vi "Curtin1_SelectTemplate.vi"(11 "Settings in":T1={"Name of test"="", "Date"=timestamp(0 s since 1904-01-01), "Location"="", "Template"="", "Soundcard"="", "resolution"=32, "Sampling rate"=48000, "Ch1 Gain "=25.0, "Ch2 Gain"=10.0, "Sample time (s)"=0.3, "Pre-trigger (s)"=0.01, "Hammer Threshold"=10.0, "Positions"=12, "Taps/Position"=5, "Set Names"="", "Freq resolution"=10.0, "Hammer cutoff"=0.0, "Mic cutoff"=0.0, "Double bounce "=0.0, "Hammer Cal"=10.0, "dB Offset"=0.0, "Accel Cal"=10.0, "Vibrometer Cal"=0.0, "Mic Cal"=0.0, "Output"=2, "Voltage Cal"=0.01, "Vibrometer Port"="ASRL27::INSTR", "Range"=4, "High Pass"=2, "Bandwidth"=4, "X Range"=[], "Y Range"=[], "dB Spread"=0.0, "Trigger"=0, "Ch_1"=25, "Ch_2"=25, "flip?"=FALSE, "60Hz"=FALSE, "Time offset"=0.0, "Piezo Cal"=1.0, "Default Notes"=""} {"Ch_2" min=1 step=1; "Ch_1" min=1 max=100 step=1; "Trigger" items=["Hammer (force)", "Self-tap", "Spacebar"]; "Bandwidth" items=["1 kHz"=1, "5 kHz"=5, "10 kHz"=10, "25 kHz"=25, "50 kHz"=50, "100 kHz"=100]; "High Pass" items=["Off", "13 Hz", "104 Hz"]; "Range" items=["10 mm/s"=1, "20 mm/s"=2, "50 mm/s"=5, "100 mm/s"=10, "200 mm/s"=20, "500 mm/s"=50, "1 m/s"=100, "2 m/s"=200]; "Output" items=["Accelerometer", "Speed (from acceleration)", "Microphone", "Vibrometer", "Piezo"]; "Voltage Cal" format="%#_13g"; "Ch2 Gain" format="%#_13g"; "Ch1 Gain" format="%#_13g"; "Double bounce" min=0.0; "Mic cutoff" min=0.0 format="%#_4g"; "Hammer cutoff" min=0.0 format="%#_4g"; "Freq resolution" min=0.0; "Pre-trigger (s)" format="%#_13g"; "Date" format="%<%H:%M\n%d/%m/%y>T"; "resolution" items=["16 bit"=16, "24 bit"=24, "32 bit"=32]; "Sampling rate" items=["22050 samp/s"=22050, "44100 samp/s"=44100, "48000 samp/s"=48000]}) -> (1 "New Template":string, 3 "Settings out":T1={"Name of test"="", "Date"=timestamp(0 s since 1904-01-01), "Location"="", "Template"="", "Soundcard"="", "resolution"=32, "Sampling rate"=48000, "Ch1 Gain "=25.0, "Ch2 Gain"=10.0, "Sample time (s)"=0.3, "Pre-trigger (s)"=0.01, "Hammer Threshold"=10.0, "Positions"=12, "Taps/Position"=5, "Set Names"="", "Freq resolution"=10.0, "Hammer cutoff"=0.0, "Mic cutoff"=0.0, "Double bounce "=0.0, "Hammer Cal"=10.0, "dB Offset"=0.0, "Accel Cal"=10.0, "Vibrometer Cal"=0.0, "Mic Cal"=0.0, "Output"=2, "Voltage Cal"=0.01, "Vibrometer Port"="ASRL27::INSTR", "Range"=4, "High Pass"=2, "Bandwidth"=4, "X Range"=[], "Y Range"=[], "dB Spread"=0.0, "Trigger"=0, "Ch_1"=25, "Ch_2"=25, "flip?"=FALSE, "60Hz"=FALSE, "Time offset"=0.0, "Piezo Cal"=1.0, "Default Notes"=""} {"Ch_2" min=1 step=1; "Ch_1" min=1 max=100 step=1; "Trigger" items=["Hammer (force)", "Self-tap", "Spacebar"]; "Bandwidth" items=["1 kHz"=1, "5 kHz"=5, "10 kHz"=10, "25 kHz"=25, "50 kHz"=50, "100 kHz"=100]; "High Pass" items=["Off", "13 Hz", "104 Hz"]; "Range" items=["10 mm/s"=1, "20 mm/s"=2, "50 mm/s"=5, "100 mm/s"=10, "200 mm/s"=20, "500 mm/s"=50, "1 m/s"=100, "2 m/s"=200]; "Output" items=["Accelerometer", "Speed (from acceleration)", "Microphone", "Vibrometer", "Piezo"]; "Voltage Cal" format="%#_13g"; "Ch2 Gain" format="%#_13g"; "Ch1 Gain" format="%#_13g"; "Double bounce" min=0.0; "Mic cutoff" min=0.0 format="%#_4g"; "Hammer cutoff" min=0.0 format="%#_4g"; "Freq resolution" min=0.0; "Pre-trigger (s)" format="%#_13g"; "Date" format="%<%H:%M\n%d/%m/%y>T"; "resolution" items=["16 bit"=16, "24 bit"=24, "32 bit"=32]; "Sampling rate" items=["22050 samp/s"=22050, "44100 samp/s"=44100, "48000 samp/s"=48000]})   [LabVIEW 2022 SP3]
uses:
  PreferencesControl.ctl
panel:
  in  "Settings File":bool
  in  "delete":bool
  in  "Cancel Button":bool
  in  "OK Button":bool
  in  "Template File":string(combo)
  in  "Edit":bool
  # "Hz"
  # "dB"
  # "dB"
  # "sec"
  # "sec"
  # "mV/Pa"
  # "mV/m/s2"
  # "mV/mm/s"
  # "V/N"
  # "sec"
  # "sec"
  # "mV/N"
  # "a.u."
  # "a.u."
  # "sec"
  # "Hz"
  # "dB"
  # "dB"
  # "sec"
  # "sec"
  # "mV/Pa"
  # "mV/m/s2"
  # "mV/mm/s"
  # "V/N"
  # "sec"
  # "sec"
  # "mV/N"
  # "a.u."
  # "a.u."
  # "sec"
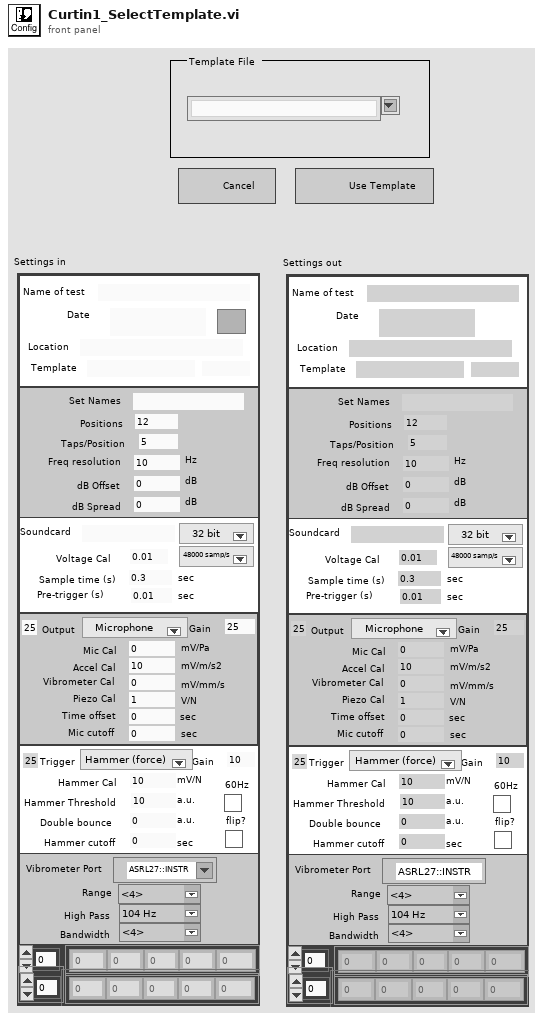
[diagram p1: front panel]
types:
  T1 = typedef "PreferencesControl.ctl" = cluster{"Name of test":string, "Date":timestamp, "Location":string, "Template":string, "Soundcard":string, "resolution":u16, "Sampling rate":u16, "Ch1 Gain ":dbl, "Ch2 Gain":dbl, "Sample time (s)":dbl, "Pre-trigger (s)":dbl, "Hammer Threshold":dbl, "Positions":i16, "Taps/Position":i16, "Set Names":string, "Freq resolution":dbl, "Hammer cutoff":dbl, "Mic cutoff":dbl, "Double bounce ":dbl, "Hammer Cal":dbl, "dB Offset":dbl, "Accel Cal":dbl, "Vibrometer Cal":dbl, "Mic Cal":dbl, "Output":u16, "Voltage Cal":dbl, "Vibrometer Port":refnum<visa-resource-name>, "Range":u16, "High Pass":u16, "Bandwidth":u16, "X Range":cluster{"Minimum":dbl, "Maximum":dbl, "Increment":dbl, "Minor Increment":dbl, "Start":dbl}[], "Y Range":cluster{"Minimum":dbl, "Maximum":dbl, "Increment":dbl, "Minor Increment":dbl, "Start":dbl}[], "dB Spread":dbl, "Trigger":u16, "Ch_1":u8, "Ch_2":u8, "flip?":bool, "60Hz":bool, "Time offset":dbl, "Piezo Cal":dbl, "Default Notes":string}
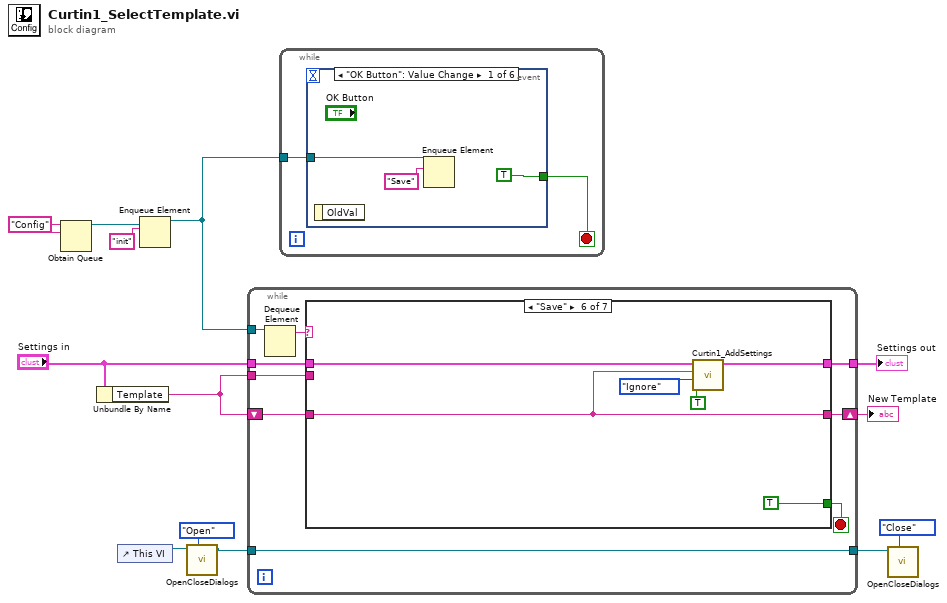
[diagram p0: block diagram]
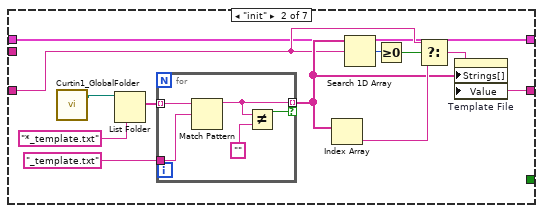
[diagram p3: hidden frame]
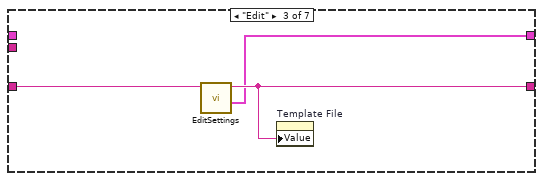
[diagram p4: hidden frame]
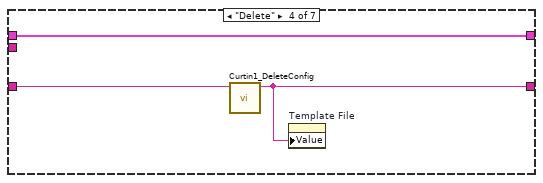
[diagram p5: hidden frame]
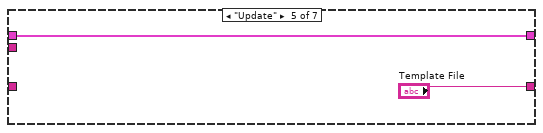
[diagram p6: hidden frame]
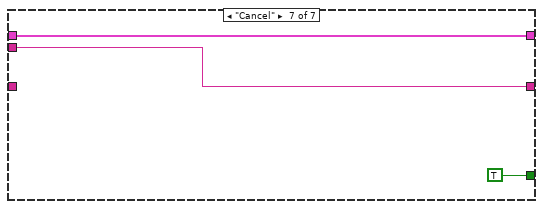
[diagram p7: hidden frame]
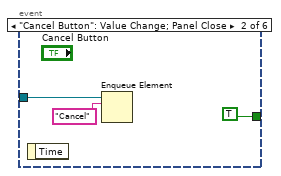
[diagram p8: hidden frame]
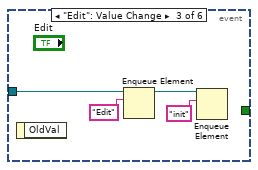
[diagram p9: hidden frame]
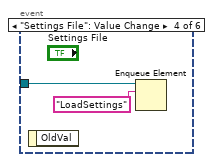
[diagram p10: hidden frame]
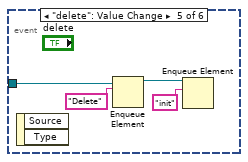
[diagram p11: hidden frame]
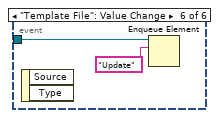
[diagram p12: hidden frame]
diagram:
  w13 = "Config" ("name (unnamed)")
  n1 = Obtain Queue(name (unnamed)=w13, element data type=w13) -> (queue out=w12:refnum<queue>)  [unwired: 3 in, 2 out]
  n2 = Unbundle By Name("Settings in") -> ("Template"=w10:string)
  n3 = control-ref of="This VI"() -> (w4:refnum<vi>)
  n4 = Enqueue Element(queue=w12, element="init") -> (queue out=w9:refnum<queue>)  [unwired: 2 in, 2 out]
  n5 = call "OpenCloseDialogs.vi"("Task"=enum16{"Open", "Close"}."Open", "VI in"=w4) -> ("VI out"=w1:refnum<vi>)  [unwired: 8 in, 1 out]
  n6 = while {
    tunnel: w9 -> [w21]
    tunnel: w10 -> [w20]
    shift-right: [w15] -> w6
    shift-left: w10 -> [w19]
    tunnel: "Settings in" -> [w17]
    tunnel: [w16] -> w7
    tunnel: [w14] -> w2
    tunnel: w1 -> [w14]
    stop <- w18 stop-if-true
    n7 = Dequeue Element(queue=w21) -> (element=w22:string)  [unwired: 2 in, 3 out]
    n8 = case shown="\"Save\"" w22 {
      tunnel: w20 -> [_ _ _ _ _ _ w57]
      tunnel: [w24 w27 w42 w45 "Template File" w51 w57] -> w15
      tunnel: w19 -> [w24 w26 w43 w46 _ w51 _]
      tunnel: [_ _ _ _ _ TRUE TRUE] -> w18
      tunnel: w17 -> [w23 w25 _ w44 w47 w53 w55]
      tunnel: [w23 w25 w41 w44 w47 w52 w55] -> w16
      frame Default {
      }
      frame "init" {
        n9 = call "Curtin1_GlobalFolder.vi"() -> ("LabVIEW Data Path"=w35:path)  [unwired: 1 in, 1 out]
        n10 = List Folder(path=w35, pattern="*_template.txt") -> (filenames=w30:string[])  [unwired: 2 in, 3 out]
        n11 = for {
          tunnel: w30 -> [w40] mode=indexing
          tunnel: [w38] -> w31 mode=indexing if=w37
          tunnel: "_template.txt" ("pattern") -> [w39]
          n12 = Match Pattern(string=w40, regular expression=w39) -> (before substring=w38:string)  [unwired: 4 out]
          n13 = Not Equal?(x=w38, y="") -> (x != y?=w37:bool)
        }
        n14 = Index Array(array=w31) -> (element=w34:string)  [unwired: 1 in]
        n15 = Search 1D Array(1D array=w31, element=w26) -> (index of element=w32:i32)  [unwired: 1 in]
        n16 = Greater Or Equal To 0?(x=w32) -> (x >= 0?=w33:bool)
        n17 = Select(t=w26, s=w33, f=w34) -> (s? t:f=w27:string)
        n18 = property on="Template File" class="CmbBox"("Strings[]"=w31, "Value"=w27) -> ()  [unwired: 2 in, 2 out]
      }
      frame "Edit" {
        n19 = call "EditSettings.vi"("Template in"=w43) -> ("Settings out"=w41:T1, "Template out"=w42:string)  [unwired: 9 in]
        n20 = property on="Template File" class="CmbBox"("Value"=w42) -> ()  [unwired: 2 in, 2 out]
      }
      frame "Delete" {
        n21 = call "Curtin1_DeleteConfig.vi"("Test Configuration"=w46) -> ("New File"=w45:string)  [unwired: 10 in]
        n22 = property on="Template File" class="CmbBox"("Value"=w45) -> ()  [unwired: 2 in, 2 out]
      }
      frame "Update" {
      }
      frame "Save" {
        n23 = call "Curtin1_AddSettings.vi"("Date?"=TRUE, "Check?"=enum16{"Ignore", "Check", "Replace"}."Ignore", "Template"=w51, "Settings in"=w53) -> ("Settings Out"=w52:T1)  [unwired: 6 in, 1 out]
      }
      frame "Cancel" {
      }
    }
  }
  "Settings out" <- w7
  "New Template" <- w6
  n24 = while {
    tunnel: w9 -> [w58]
    stop <- w59 stop-if-true
    n25 = event shown="[0] \"OK Button\": Value Change" {
      selector: _ -> [_ _ _ _ _ _]
      dyn-events: _ -> [_ _ _ _ _ _]
      timeout: _ -> [_ _ _ _ _ _]
      tunnel: [TRUE ("OK Button") TRUE ("OK Button") _ _ _ _] -> w59
      tunnel: w58 -> [w60 w63 w68 w70 w74 w76]
      event "OK Button": Value Change {
        n26 = event-data() -> ()  [unwired: 1 in, 1 out]
        n27 = Enqueue Element(queue=w60, element="Save") -> ()  [unwired: 2 in, 3 out]
      }
      event "Cancel Button": Value Change; Panel Close {
        n28 = event-data() -> ()  [unwired: 1 in, 1 out]
        n29 = Enqueue Element(queue=w63, element="Cancel") -> ()  [unwired: 2 in, 3 out]
      }
      event "Edit": Value Change {
        n30 = event-data() -> ()  [unwired: 1 in, 1 out]
        n31 = Enqueue Element(queue=w68, element="Edit") -> (queue out=w66:refnum<queue>)  [unwired: 2 in, 2 out]
        n32 = Enqueue Element(queue=w66, element="init") -> ()  [unwired: 2 in, 3 out]
      }
      event "Settings File": Value Change {
        n33 = event-data() -> ()  [unwired: 1 in, 1 out]
        n34 = Enqueue Element(queue=w70, element="LoadSettings") -> ()  [unwired: 2 in, 3 out]
      }
      event "delete": Value Change {
        n35 = event-data() -> ()  [unwired: 1 in, 2 out]
        n36 = Enqueue Element(queue=w74, element="Delete") -> (queue out=w72:refnum<queue>)  [unwired: 2 in, 2 out]
        n37 = Enqueue Element(queue=w72, element="init") -> ()  [unwired: 2 in, 3 out]
      }
      event "Template File": Value Change {
        n38 = event-data() -> ()  [unwired: 1 in, 2 out]
        n39 = Enqueue Element(queue=w76, element="Update") -> ()  [unwired: 2 in, 3 out]
      }
    }
  }
  n40 = call "OpenCloseDialogs.vi"("Task"=enum16{"Open", "Close"}."Close", "VI in"=w2) -> ()  [unwired: 8 in, 2 out]
